vi "Package Details URL--constant.vi"() -> (3 "Package Details URL":string="https://intranet.studiobods.com/public/temp/GCentral/PackageDetails.html")   [LabVIEW 2016, in "WSsupport.lvlib"]
uses:
  WSsupport.lvlib
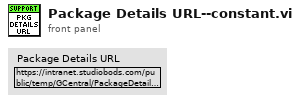
[diagram p1: front panel]
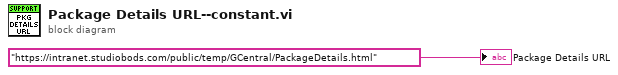
[diagram p0: block diagram]
diagram:
  "Package Details URL" <- "https://intranet.studiobods.com/public/temp/GCentral/PackageDetails.html"
